vi "isLevel.vi"(9 "IO Module\\DDCA_DIO0_Write":bool, 10 "State":i32, 11 "Divider_Sclk":i32) -> (2 "Level":enum16{"Else", "Low", "High"}(ring))   [LabVIEW 2018]
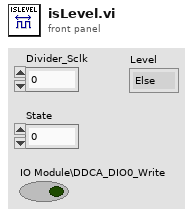
[diagram p1: front panel]
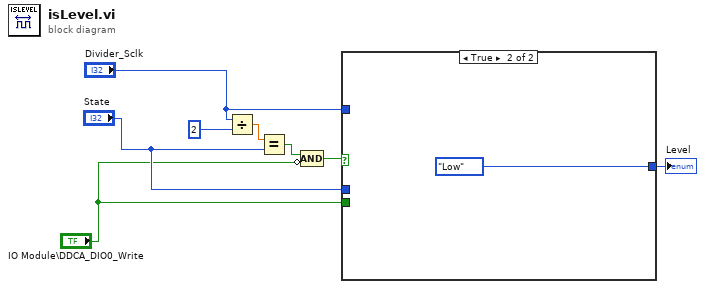
[diagram p0: block diagram]
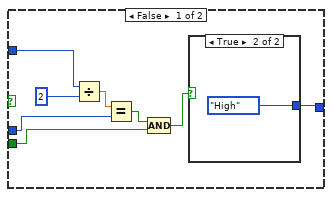
[diagram p2: hidden frame]
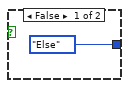
[diagram p3: hidden frame]
diagram:
  n1 = Divide(x="Divider_Sclk", y=2) -> (x/y=w8:dbl)
  n2 = Equal?(x=w8, y="State") -> (x = y?=w6:bool)
  n3 = Compound Arithmetic op=AND(w6, invert "IO Module\\DDCA_DIO0_Write") -> (w5:bool)
  n4 = case shown="True" w5 {
    tunnel: [w9 enum16{"Else", "Low", "High"}."Low"] -> w1
    tunnel: "Divider_Sclk" -> [w13 _]
    tunnel: "State" -> [w12 _]
    tunnel: "IO Module\\DDCA_DIO0_Write" -> [w11 _]
    frame False {
      n5 = Divide(x=w13, y=2) -> (x/y=w14:dbl)
      n6 = Equal?(x=w14, y=w12) -> (x = y?=w16:bool)
      n7 = Compound Arithmetic op=AND(w16, w11) -> (w10:bool)
      n8 = case shown="True" w10 {
        tunnel: [enum16{"Else", "Low", "High"}."Else" enum16{"Else", "Low", "High"}."High"] -> w9
        frame False {
        }
        frame True {
        }
      }
    }
    frame True {
    }
  }
  "Level" <- w1
